vi "_Simple_Demo.vi"() -> ()   [LabVIEW 2022 SP3]
uses:
  Processors.ctl
panel:
  out "Version":string
  out "Port":string
  out "Data":dbl[](graph)
  out "Image":picture
  in  "stop":bool
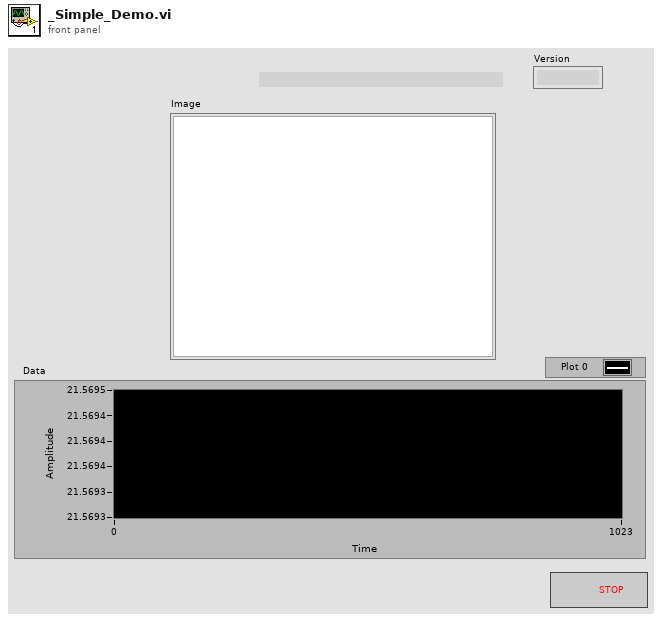
[diagram p1: front panel]
types:
  T1 = typedef "Processors.ctl" = enum16{"SPIKE", "Pi", "Pi_ssh", "OpenMV", "Dunio"}
  T2 = typedef "Preferences.ctl" = cluster{"python":string, "arduino CLI":path, "pythonCodes":cluster{"pythonCode":path, "Color":u32}[], "FontSize":u8, "Text Colors":cluster{"Quote":u32, "function":u32, "Python":u32, "Comment":u32, "Triple Quote":u32, "Text":u32}, "SSH Logins":cluster{"IP Address":string, "Username":string, "password":string}[], "packet size":u8}
  T3 = typedef "PythonCtrl.ctl" = cluster{"session":refnum<k35>, "PyPath":path, "Processor":T1, "Port":string, "version":string}
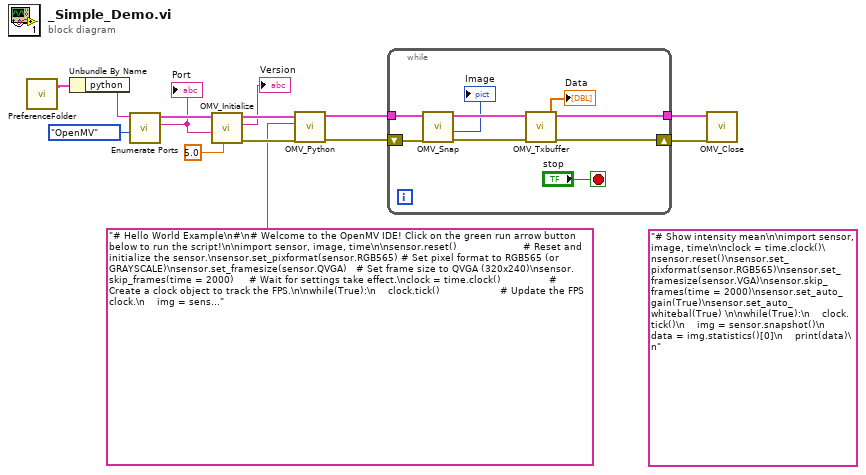
[diagram p0: block diagram]
diagram:
  (unwired) "# Show intensity mean\n\nimport sensor, image, time\n\nclock = time.clock()\nsensor.reset()\nsensor.set_pixformat(sensor.RGB565)\nsensor.set_framesize(sensor.VGA)\nsensor.skip_frames(time = 2000)\nsensor.set_auto_gain(True)\nsensor.set_auto_whitebal(True) \n\nwhile(True):\n    clock.tick()\n    img = sensor.snapshot()\n    data = img.statistics()[0]\n    print(data)\n"
  n1 = call "PreferenceFolder.vi"() -> ("Everything"=w2:T2)  [unwired: 4 in, 7 out]
  n2 = Unbundle By Name(w2) -> ("python"=w1:string)
  n3 = call "Enumerate Ports.vi"("Processor"=Processors."OpenMV", "Python version"=w1) -> ("Short guess"=w3:string, "Python"=w12:T3)  [unwired: 4 in, 4 out]
  "Port" <- w3
  n4 = call "OMV_Initialize.vi"("timeout"=5.0, "Port"=w3, "Python"=w12) -> ("error out"=w9:errorcluster, "Version"=→"Version":string, "Python"=w7:T3)  [unwired: 6 in]
  n5 = call "OMV_Python.vi"("error in (no error)"=w9, "Script"="# Hello World Example\n#\n# Welcome to the OpenMV IDE! Click on the green run arrow button below to run the script!\n\nimport sensor, image, time\n\nsensor.reset()                      # Reset and initialize the sensor.\nsensor.set_pixformat(sensor.RGB565) # Set pixel format to RGB565 (or GRAYSCALE)\nsensor.set_framesize(sensor.QVGA)   # Set frame size to QVGA (320x240)\nsensor.skip_frames(time = 2000)     # Wait for settings take effect.\nclock = time.clock()                # Create a clock object to track the FPS.\n\nwhile(True):\n    clock.tick()                    # Update the FPS clock.\n    img = sensor.snapshot()         # Take a picture and return the image.\n    print(clock.fps())              # Note: OpenMV Cam runs about half as fast when connected\n                                    # to the IDE. The FPS should increase once disconnected.\n", "Python"=w7) -> ("error out"=w10:errorcluster, "Python"=w6:T3)  [unwired: 7 in]
  n6 = while {
    tunnel: w6 -> [w23]
    tunnel: [w21] -> w14
    shift-right: [w18] -> w11
    shift-left: w10 -> [w16]
    stop <- "stop" stop-if-true
    n7 = call "OMV_Snap.vi"("error in (no error)"=w16, "Python"=w23) -> ("error out"=w19:errorcluster, "picture"=→"Image":picture, "Python"=w22:T3)  [unwired: 6 in, 1 out]
    n8 = call "OMV_Txbuffer.vi"("error in (no error)"=w19, "Python"=w22) -> ("error out"=w18:errorcluster, "Data"=→"Data":dbl[], "Python"=w21:T3)  [unwired: 7 in]
  }
  n9 = call "OMV_Close.vi"("error in (no error)"=w11, "Python"=w14) -> ()  [unwired: 10 in]
